vi "joystick interpreter.vi"(8 "error in (no error)":errorcluster, 11 "Refnum in":refnum<k1>) -> (0 "error out":errorcluster, 1 "v_tang":dbl format="%0.2f", 2 "v_norm":dbl format="%0.2f", 3 "Refnum out":refnum<k1>, 4 "v_ang":dbl format="%0.2f")   [LabVIEW 2020]
uses:
  <vilib>/ptbypt/NI_PtbyPt.lvlib
panel:
  out "X axis rotation":i32
  out "Y axis":i32
  out "Y axis rotation":i32
  out "Z axis":i32
  out "pov 1":i32
  out "X axis":i32
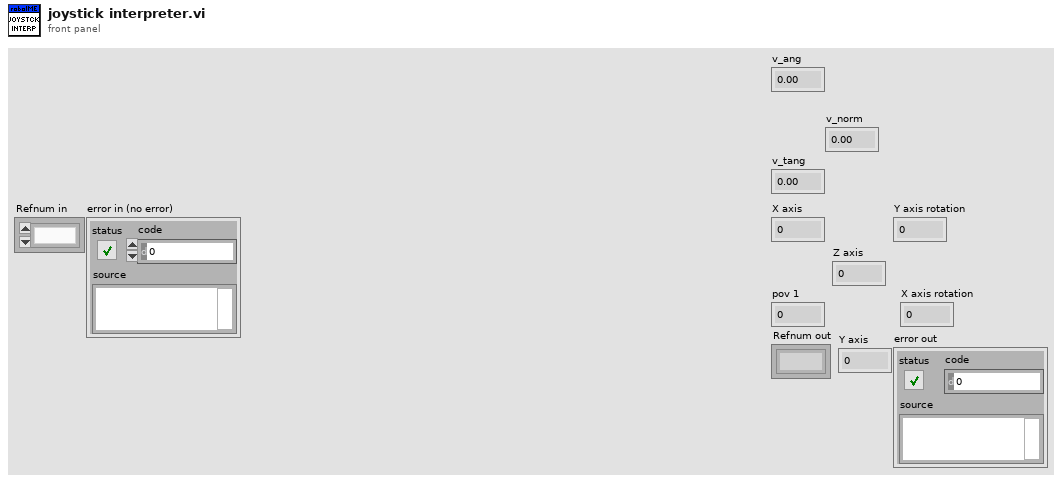
[diagram p1: front panel]
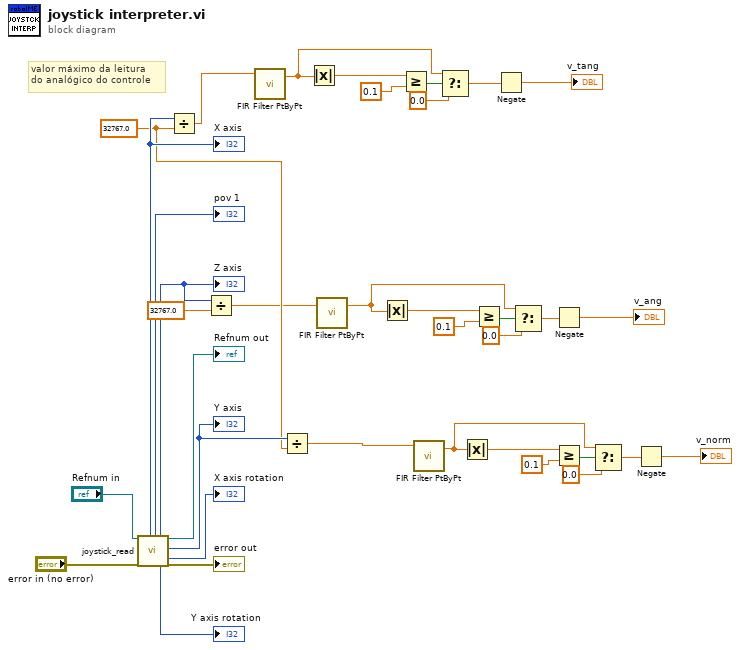
[diagram p0: block diagram]
diagram:
  w26 = 32767.0
  # "valor máximo da leitura\ndo analógico do controle"
  n1 = call "joystick_read.vi"("Refnum in"="Refnum in", "error in (no error)"="error in (no error)") -> ("X axis"=w29:i32, "pov 1"=→"pov 1":i32, "Z axis"=w14:i32, "Y axis rotation"=→"Y axis rotation":i32, "Refnum out"=→"Refnum out":refnum<k1>, "Y axis"=w27:i32, "X axis rotation"=→"X axis rotation":i32, "error out"=→"error out":errorcluster)  [unwired: 6 in, 4 out]
  "X axis" <- w29
  "Z axis" <- w14
  "Y axis" <- w27
  n2 = Divide(x=w29, y=w26) -> (x/y=w28:dbl)
  n3 = Divide(x=w14, y=32767.0) -> (x/y=w13:dbl)
  n4 = call <vilib>:"FIR Filter PtByPt.vi"("x"=w28) -> ("Filtered x"=w21:dbl)  [unwired: 3 in, 1 out]
  n5 = Divide(x=w27, y=w26) -> (x/y=w7:dbl)
  n6 = Absolute Value(x=w21) -> (abs(x)=w22:dbl)
  n7 = call <vilib>:"FIR Filter PtByPt.vi"("x"=w13) -> ("Filtered x"=w8:dbl)  [unwired: 3 in, 1 out]
  n8 = Absolute Value(x=w8) -> (abs(x)=w9:dbl)
  n9 = Greater Or Equal?(x=w22, y=0.1) -> (x >= y?=w24:bool)
  n10 = call <vilib>:"FIR Filter PtByPt.vi"("x"=w7) -> ("Filtered x"=w16:dbl)  [unwired: 3 in, 1 out]
  n11 = Select(t=w21, s=w24, f=0.0) -> (s? t:f=w6:dbl)
  n12 = Absolute Value(x=w16) -> (abs(x)=w17:dbl)
  n13 = Greater Or Equal?(x=w9, y=0.1) -> (x >= y?=w11:bool)
  n14 = Negate(x=w6) -> (-x=→"v_tang":dbl)
  n15 = Select(t=w8, s=w11, f=0.0) -> (s? t:f=w2:dbl)
  n16 = Negate(x=w2) -> (-x=→"v_ang":dbl)
  n17 = Greater Or Equal?(x=w17, y=0.1) -> (x >= y?=w19:bool)
  n18 = Select(t=w16, s=w19, f=0.0) -> (s? t:f=w4:dbl)
  n19 = Negate(x=w4) -> (-x=→"v_norm":dbl)
